vi "average data.vi"(6 "state":T6=enum."Change setpoints", 8 "error in (no error)":errorcluster, 9 "setpoints":T2={"graph data interval (s)"=100.0, "sludge flow [L/s]"=0.0, "plant flow [L/s]"=0.05, "Plant Flow PID "={"proportional gain (Kc)"=0.05, "integral time (Ti, min)"=1.0, "derivative time (Td, min)"=0.01}, "Sludge PID "={"proportional gain (Kc)"=0.07, "integral time (Ti, min)"=1.0, "derivative time (Td, min)"=0.01}, "backwash"={"Filtered quality target [NTU]"=0.3, "min filtration time [s]"=600.0, "Ripen time [s]"=600.0}, "Coagulant"={"flocculator volume (L)"=0.0, "clarifier volume (L)"=0.0, "dose updates per HRT"=1, "target clarified turbidity (NTU)"=0.3, "Coagulant mode"=enum."Manual", "Coag dose [mg/L]"=0.0}} {"Coagulant"."target clarified turbidity (NTU)" min=0.1 max=5.0 step=0.01; "Coagulant"."dose updates per HRT" min=1 max=1000 step=1; "Sludge PID"."derivative time (Td, min)" format="%.3f"; "Sludge PID"."integral time (Ti, min)" format="%.3f"; "Sludge PID"."proportional gain (Kc)" format="%.3f"; "Plant Flow PID"."derivative time (Td, min)" format="%.3f"; "Plant Flow PID"."integral time (Ti, min)" format="%.3f"; "Plant Flow PID"."proportional gain (Kc)" format="%.3f"; "plant flow [L/s]" min=0.05 max=1.0 step=0.05; "sludge flow [L/s]" min=0.0 max=0.05 step=0.001; "graph data interval (s)" min=1 max=1000 step=1}, 10 "data input":dbl[](array[numeric])) -> (0 "error out":errorcluster, 1 "new interval":bool, 2 "averaged data":T7, 3 "total HRT":dbl, 4 "coag model":T1)   [LabVIEW 2015]
uses:
  setpoints.ctl
  backwash.ctl
  coag.ctl
  Manual or Auto.ctl
  data array with time.ctl
  data ave state.ctl
  model type.ctl
  Sensor buffer command.ctl
  data channels.ctl
  state.ctl
panel:
  out "setpoints out":T2={"graph data interval (s)"=100.0, "sludge flow [L/s]"=0.0, "plant flow [L/s]"=0.05, "Plant Flow PID "={"proportional gain (Kc)"=0.05, "integral time (Ti, min)"=1.0, "derivative time (Td, min)"=0.01}, "Sludge PID "={"proportional gain (Kc)"=0.07, "integral time (Ti, min)"=1.0, "derivative time (Td, min)"=0.01}, "backwash"={"Filtered quality target [NTU]"=0.3, "min filtration time [s]"=600.0, "Ripen time [s]"=600.0}, "Coagulant"={"flocculator volume (L)"=0.0, "clarifier volume (L)"=0.0, "dose updates per HRT"=100, "target clarified turbidity (NTU)"=0.3, "Coagulant mode"=enum."Manual", "Coag dose [mg/L]"=0.0}} {"Coagulant"."target clarified turbidity (NTU)" min=0.1 max=5.0 step=0.01; "Coagulant"."dose updates per HRT" min=1 max=1000 step=1; "Sludge PID"."derivative time (Td, min)" format="%.3f"; "Sludge PID"."integral time (Ti, min)" format="%.3f"; "Sludge PID"."proportional gain (Kc)" format="%.3f"; "Plant Flow PID"."derivative time (Td, min)" format="%.3f"; "Plant Flow PID"."integral time (Ti, min)" format="%.3f"; "Plant Flow PID"."proportional gain (Kc)" format="%.3f"; "plant flow [L/s]" min=0.05 max=1.0 step=0.05; "sludge flow [L/s]" min=0.0 max=0.05 step=0.001; "graph data interval (s)" min=1 max=1000 step=1}
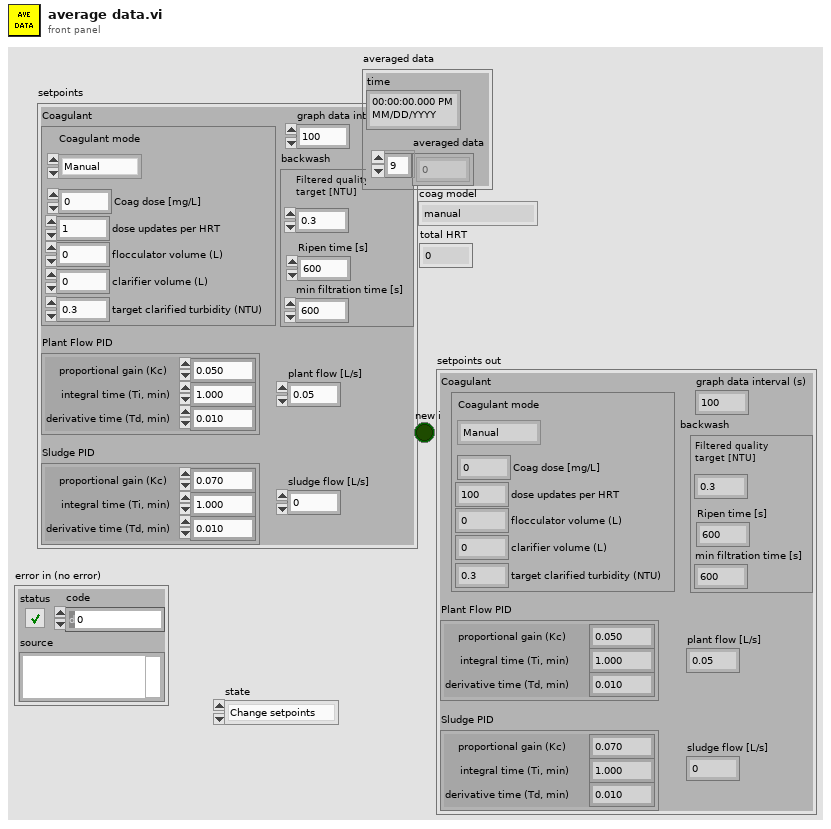
[diagram p1: front panel]
types:
  T1 = typedef "model type.ctl" = enum16{"manual", "simple corrector", "linear regression"}
  T2 = typedef "setpoints.ctl" = cluster{"graph data interval (s)":sgl, "sludge flow [L/s]":dbl, "plant flow [L/s]":dbl, "Plant Flow PID ":cluster{"proportional gain (Kc)":dbl, "integral time (Ti, min)":dbl, "derivative time (Td, min)":dbl}, "Sludge PID ":cluster{"proportional gain (Kc)":dbl, "integral time (Ti, min)":dbl, "derivative time (Td, min)":dbl}, "backwash":T3, "Coagulant":T4}
  T3 = typedef "backwash.ctl" = cluster{"Filtered quality target [NTU]":dbl, "min filtration time [s]":dbl, "Ripen time [s]":dbl}
  T4 = typedef "coag.ctl" = cluster{"flocculator volume (L)":dbl, "clarifier volume (L)":dbl, "dose updates per HRT":u32, "target clarified turbidity (NTU)":dbl, "Coagulant mode":T5, "Coag dose [mg/L]":dbl}
  T5 = typedef "Manual or Auto.ctl" = enum16{"Manual", "Automatic"}
  T6 = typedef "data ave state.ctl" = enum16{"Initialize", "Change setpoints", "Process data"}
  T7 = typedef "data array with time.ctl" = cluster{"time":timestamp, "averaged data":dbl[]}
  T8 = typedef "Sensor buffer command.ctl" = enum16{"set buffer size", "write", "refill buffer", "read recent", "read all", "clear"}
  T9 = typedef "state.ctl" = enum16{"Initialize", "Change setpoints", "Process data", "Close"}
  T10 = typedef "data channels.ctl" = enum16{"plant flow [L/s]", "Head Loss [m]", "sludge flow [L/s]", "UV 254", "raw [NTU]", "floc [NTU]", "clarified [NTU]", "filtered [NTU]"}
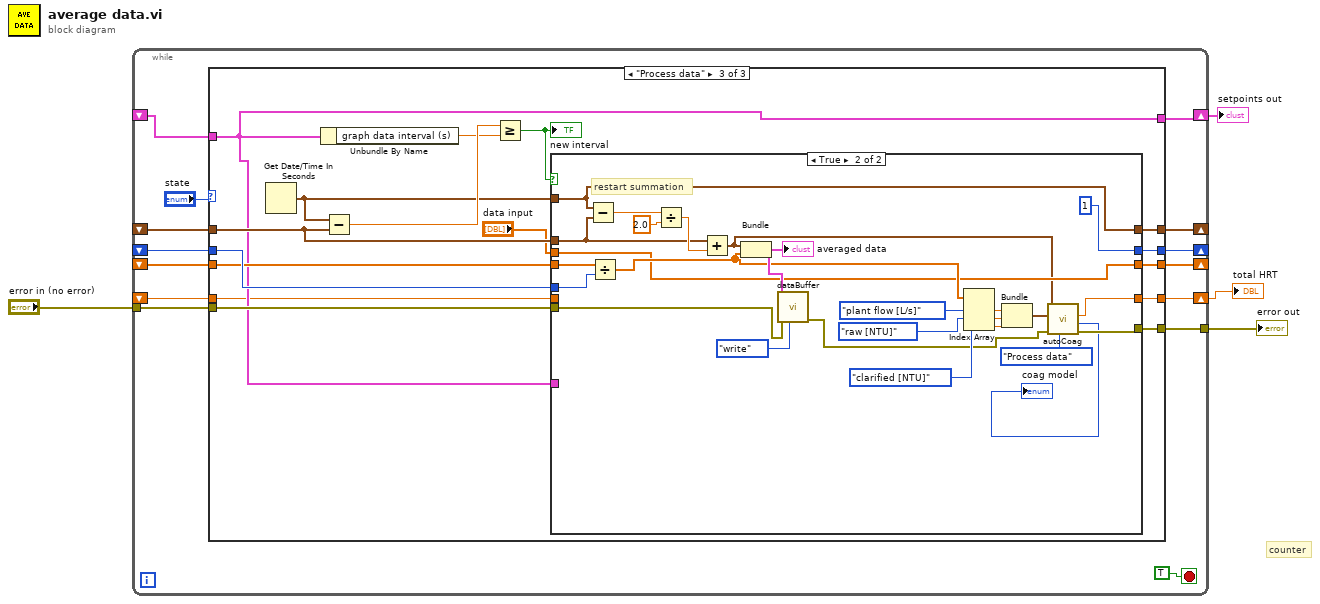
[diagram p0: block diagram]
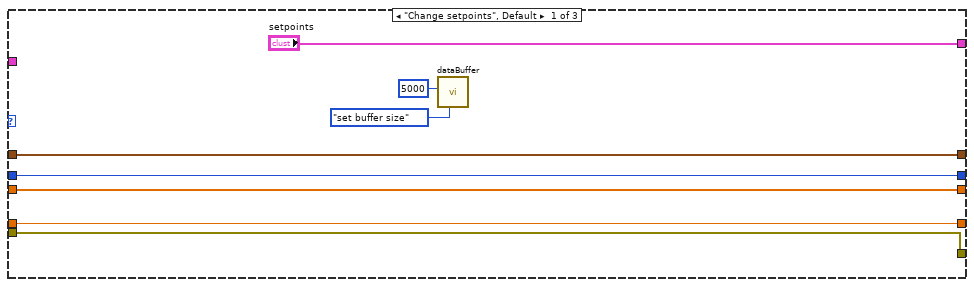
[diagram p2: hidden frame]
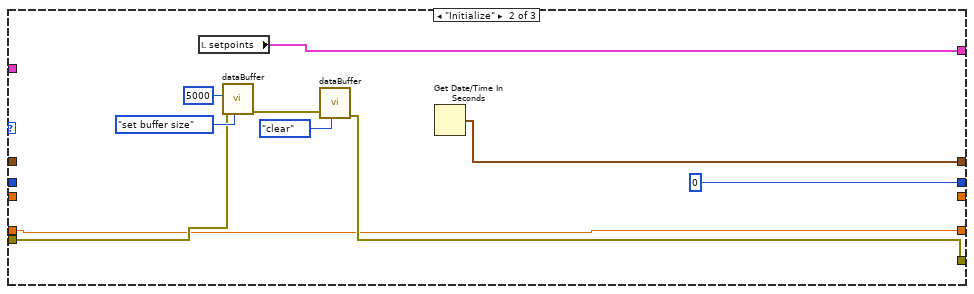
[diagram p3: hidden frame]
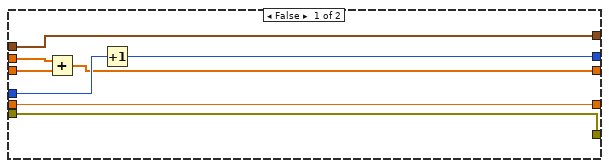
[diagram p4: hidden frame]
diagram:
  # "counter"
  n1 = while {
    shift-right: [w15] -> _
    shift-left: _ -> [w12]
    shift-right: [w17] -> _
    shift-left: _ -> [w16]
    shift-right: [w14] -> _
    shift-left: _ -> [w13]
    shift-right: [w10] -> w4
    shift-left: _ -> [w9]
    tunnel: "error in (no error)" -> [w8]
    tunnel: [w7] -> w2
    shift-right: [w6] -> w1
    shift-left: _ -> [w5]
    stop <- TRUE stop-if-true
    n2 = case shown="\"Process data\"" "state" {
      tunnel: [w24 0 w52] -> w17
      tunnel: w16 -> [w24 _ w51]
      tunnel: [w25 w35 w50] -> w15
      tunnel: [w23 _ w49] -> w14
      tunnel: w13 -> [w23 _ w48]
      tunnel: w12 -> [w25 _ w47]
      tunnel: ["setpoints" w36 w39] -> w10
      tunnel: w9 -> [_ _ w39]
      tunnel: [w22 w28 w40] -> w7
      tunnel: w8 -> [w22 w29 w41]
      tunnel: [w19 w27 w38] -> w6
      tunnel: w5 -> [w19 w27 w37]
      frame "Change setpoints", Default {
        n3 = call "dataBuffer.vi"("command"=Sensor_buffer_command."set buffer size", "max array size"=u16 5000) -> ()  [unwired: 5 in, 5 out]
      }
      frame "Initialize" {
        n4 = local read "setpoints"() -> (w36:T2)
        n5 = call "dataBuffer.vi"("command"=Sensor_buffer_command."set buffer size", "error in (no error)"=w29, "max array size"=u16 5000) -> ("error out"=w30:errorcluster)  [unwired: 4 in, 4 out]
        n6 = call "dataBuffer.vi"("command"=Sensor_buffer_command."clear", "error in (no error)"=w30) -> ("error out"=w28:errorcluster)  [unwired: 5 in, 4 out]
        n7 = Get Date/Time In Seconds() -> (seconds since 1Jan1904=w35:timestamp)
      }
      frame "Process data" {
        n8 = Get Date/Time In Seconds() -> (seconds since 1Jan1904=w42:timestamp)
        n9 = Unbundle By Name(w39) -> ("graph data interval (s)"=w45:sgl)
        n10 = Subtract(x=w42, y=w47) -> (x-y=w46:dbl)
        n11 = Greater Or Equal?(x=w46, y=w45) -> (x >= y?=w44:bool)
        "new interval" <- w44
        n12 = case shown="True" w44 {
          tunnel: [w59 1] -> w52
          tunnel: w51 -> [w60 w80]
          tunnel: [w58 w79] -> w50
          tunnel: w42 -> [_ w79]
          tunnel: w47 -> [w58 w81]
          tunnel: [w56 w74] -> w49
          tunnel: w48 -> [w57 w85]
          tunnel: "data input" -> [w55 w74]
          tunnel: w41 -> [w54 w76]
          tunnel: [w54 w63] -> w40
          tunnel: w39 -> [_ _]
          tunnel: [w53 w61] -> w38
          tunnel: w37 -> [w53 _]
          frame False {
            n13 = Add(x=w55, y=w57) -> (x+y=w56:dbl[])
            n14 = Increment(x=w60) -> (x+1=w59:i32)
          }
          frame True {
            # "restart summation"
            n15 = Subtract(x=w79, y=w81) -> (x-y=w83:dbl)
            n16 = Divide(x=w85, y=w80) -> (x/y=w75:dbl[])
            n17 = Divide(x=w83, y=2.0) -> (x/y=w82:dbl)
            n18 = Add(x=w81, y=w82) -> (x+y=w65:timestamp)
            n19 = Bundle(w65, w75) -> (w78:cluster{timestamp, dbl[]})  [unwired: 1 in]
            "averaged data" <- w78
            n20 = call "dataBuffer.vi"("command"=Sensor_buffer_command."write", "error in (no error)"=w76, "averaged data"=w78) -> ("error out"=w64:errorcluster)  [unwired: 4 in, 4 out]
            n21 = Index Array(array=w75, index #1=data_channels."plant flow [L/s]" ("channel"), index #2=data_channels."raw [NTU]" ("channel"), index #3=data_channels."clarified [NTU]" ("channel")) -> (element #1=w73:dbl, element #2=w72:dbl, element #3=w71:dbl)
            n22 = Bundle(w73, w72, w71) -> (w66:cluster{dbl, dbl, dbl})  [unwired: 1 in]
            n23 = call "autoCoag.vi"("state"=state."Process data", "current time"=w65, "error in (no error)"=w64, "data input"=w66) -> ("error out"=w63:errorcluster, "coag model"=→"coag model":T1, "total HRT"=w61:dbl)  [unwired: 4 in, 1 out]
          }
        }
      }
    }
  }
  "error out" <- w2
  "setpoints out" <- w4
  "total HRT" <- w1
